vi "Get Version Name.vi"() -> (0 "Version Name":string)   [LabVIEW 2013]
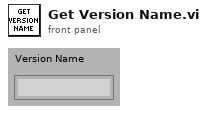
[diagram p1: front panel]
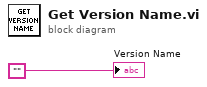
[diagram p0: block diagram]
diagram:
  "Version Name" <- "" ("Version")
